vi "Map Channel Info to VS Channels.vi"(8 "Transfer Type":string, 9 "Rx Channel Number":i32, 10 "2D Array - Label/Param List":i32[][](array[numeric])=[[1, 1], [3, 1], [3, 2], [6, 1], [8, 1], [0, 0], [0, 0], [0, 0], [0, 0], [0, 0]], 11 "VS Channel Base Port":string) -> (0 "Tx Trigger Channels Array":string[](array[string]), 1 "Tx Disable Channels Array":string[](array[string]), 2 "Tx Channels Array":string[](array[string]), 3 "Rx Channels Array":string[](array[string]))   [LabVIEW 2020, in "Single Board Loopback.lvclass"]
uses:
  Single Board Loopback.lvclass
  b281cc4c-f5bf-4263-a2a4-b8c933cd51f6.vi
  9ae52f1a-1e4b-4aa8-8e73-03c214062afe.vi
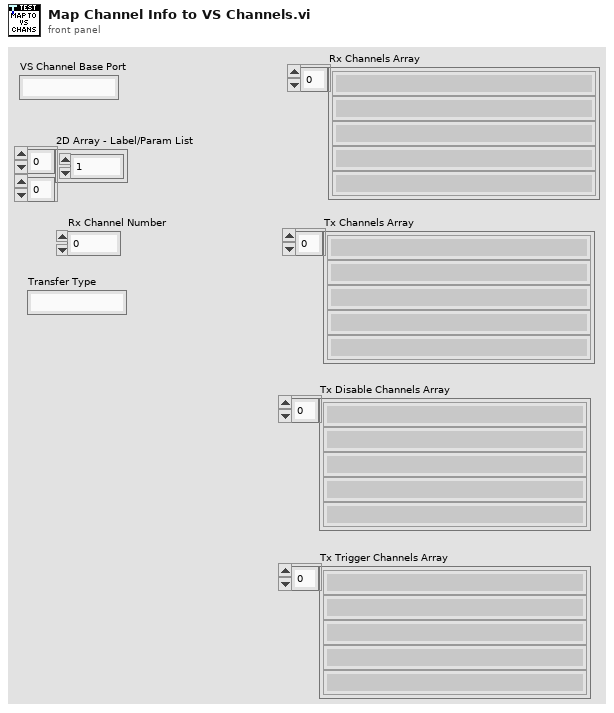
[diagram p1: front panel]
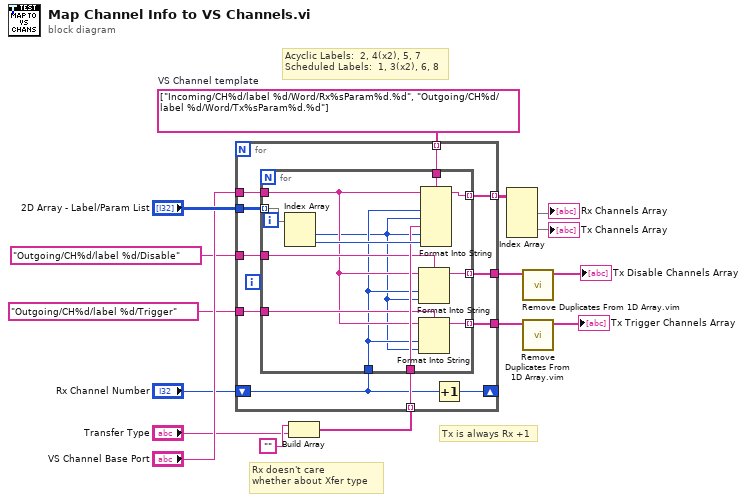
[diagram p0: block diagram]
diagram:
  w14 = string[] ["Incoming/CH%d/label %d/Word/Rx%sParam%d.%d", "Outgoing/CH%d/label %d/Word/Tx%sParam%d.%d"]  # VS Channel template
  # "Rx doesn't care\nwhether about Xfer type"
  # "Tx is always Rx +1"
  # "Acyclic Labels:  2, 4(x2), 5, 7\nScheduled Labels:  1, 3(x2), 6, 8"
  n1 = Build Array("", "Transfer Type") -> (w8:string[])
  n2 = for {
    tunnel: [w27] -> w13 mode=indexing
    tunnel: "2D Array - Label/Param List" -> [w26]
    tunnel: "VS Channel Base Port" -> [w25]
    tunnel: w14 -> [w24] mode=indexing
    tunnel: w8 -> [w23] mode=indexing
    shift-right: [w22] -> _
    shift-left: "Rx Channel Number" -> [w21]
    tunnel: "Outgoing/CH%d/label %d/Disable" ("String") -> [w20]
    tunnel: [w19] -> w2
    tunnel: "Outgoing/CH%d/label %d/Trigger" ("String") -> [w18]
    tunnel: [w17] -> w4
    n3 = for {
      tunnel: w26 -> [w39] mode=indexing
      tunnel: w24 -> [w37]
      tunnel: [w36] -> w27 mode=indexing
      tunnel: w25 -> [w31]
      tunnel: w23 -> [w35]
      tunnel: w21 -> [w30]
      tunnel: w20 -> [w34]
      tunnel: [w33] -> w19 mode=indexing
      tunnel: w18 -> [w32]
      tunnel: [w28] -> w17 mode=indexing
      n4 = Index Array(array=w39) -> (element #1=w29:i32, element #2=w38:i32)  [unwired: 2 in]
      n5 = Format Into String(format string=w34, initial string=w31, w30, w29) -> (resulting string=w33:string)  [unwired: 1 in, 1 out]
      n6 = Format Into String(format string=w32, initial string=w31, w30, w29) -> (resulting string=w28:string)  [unwired: 1 in, 1 out]
      n7 = Format Into String(format string=w37, initial string=w31, w30, w29, w35, w29, w38) -> (resulting string=w36:string)  [unwired: 1 in, 1 out]
    }
    n8 = Increment(x=w21) -> (x+1=w22:i32)
  }
  n9 = Index Array(array=w13) -> (element #1=→"Rx Channels Array":string[], element #2=→"Tx Channels Array":string[])  [unwired: 4 in]
  n10 = call "Remove Duplicates From 1D Array.vim"("array"=w2) -> ("array with duplicates removed"=→"Tx Disable Channels Array":string[])  [unwired: 10 in]
  n11 = call "Remove Duplicates From 1D Array.vim"("array"=w4) -> ("array with duplicates removed"=→"Tx Trigger Channels Array":string[])  [unwired: 10 in]
